vi "ReadTables1212(Host).vi"(0 "resource name":T1="RIO0" caption="RIO Device", 1 "Degree Offset":u16, 2 "NumSamples":u32=2048, 3 "DDS/ARB":bool=TRUE, 4 "Select Channel":u16(ring) items=["CH1", "CH2"], 5 "error in":errorcluster, 6 "FSampleDAC":dbl=2000000000.0 format="%#_6p", 7 "FoutDDS":dbl=85000000.0 format="%#_6p") -> (8 "error out":errorcluster)   [LabVIEW 2018]
uses:
  <vilib>/userdefined/High Color/nirio_resource_hc.ctl
  <vilib>/Utility/error.llb/Error Cluster From Error Code.vi
  <vilib>/rvi/errors/niLvFpgaAdjustHostInterfaceError.vi
  <vilib>/FPGAPlugInAG/Dynamic/niLvFpga_Close_Dynamic.vi
  <vilib>/rvi/interface/nirviReadWriteControl/nirviReadWriteControl.xnode
  <vilib>/rvi/interface/nirviCloseFPGA/nirviCloseFPGA.xnode
  NiFpgaLv.dll
  <vilib>/rvi/interface/Simulation/niFpgaSimulationCallBeginRW.vi
panel:
  out "FPGA Interface Out":refnum<k20>
  in  "FPGA Interface In":refnum<k20>
  in  "FLEX RIO RESET":bool
  in  "StartAddress8_CH1":u32=2920577760
  in  "StartAddress7_CH1":u32=2738041650
  in  "StartAddress6_CH1":u32=2555505540
  in  "StartAddress5_CH1":u32=2372969430
  in  "StartAddress4_CH1":u32=2190433320
  in  "StartAddress3_CH1":u32=2007897210
  in  "StartAddress2_CH1":u32=1825361100
  in  "StartAddress1_CH1":u32=1642824990
  in  "StartAddress8_CH0":u32=1460288880
  in  "StartAddress7_CH0":u32=1277752770
  in  "StartAddress6_CH0":u32=1095216660
  in  "StartAddress5_CH0":u32=912680550
  in  "StopAddress8_CH1":u32=2047
  out "Data16":fxp<+,14,14>=2760.0
  out "Data15":fxp<+,14,14>=3625.0
  in  "StopAddress7_CH1":u32=2046
  out "Data14":fxp<+,14,14>=4813.0
  in  "StopAddress6_CH1":u32=2045
  out "Data13":fxp<+,14,14>=6240.0
  in  "StopAddress5_CH1":u32=2044
  out "Data12":fxp<+,14,14>=7806.0
  in  "StopAddress4_CH1":u32=2043
  out "Data11":fxp<+,14,14>=9399.0
  in  "StopAddress3_CH1":u32=2042
  out "Data10":fxp<+,14,14>=10906.0
  out "Data9":fxp<+,14,14>=12221.0
  in  "StopAddress1_CH1":u32=2040
  in  "StopAddress2_CH1":u32=2041
  out "Data5":fxp<+,14,14>=14030.0
  in  "StopAddress5_CH0":u32=2036
  out "Data6":fxp<+,14,14>=14189.0
  in  "StopAddress6_CH0":u32=2037
  out "Data7":fxp<+,14,14>=13923.0
  in  "StopAddress7_CH0":u32=2038
  out "Data8":fxp<+,14,14>=13251.0
  in  "StopAddress8_CH0":u32=2039
  out "Data4":fxp<+,14,14>=13457.0
  out "Data3":fxp<+,14,14>=12512.0
  in  "StopAddress4_CH0":u32=2035
  in  "StopAddress3_CH0":u32=2034
  in  "StartAddress4_CH0":u32=730144440
  in  "StartAddress3_CH0":u32=547608330
  in  "Increment":u32=16 format="%.0x"
  in  "StartAddress2_CH0":u32=365072220
  in  "StopAddress2_CH0":u32=2033
  in  "StopAddress1_CH0":u32=2032
  in  "StartAddress1_CH0":u32=182536110
  in  "FPGA RESET":bool
  in  "IO Module\\trig_out":bool
  out "IO Module\\lockedfast":bool=TRUE
  out "IO Module\\trig_in":bool
  out "Data2":fxp<+,14,14>=11261.0
  out "Data1":fxp<+,14,14>=9792.0
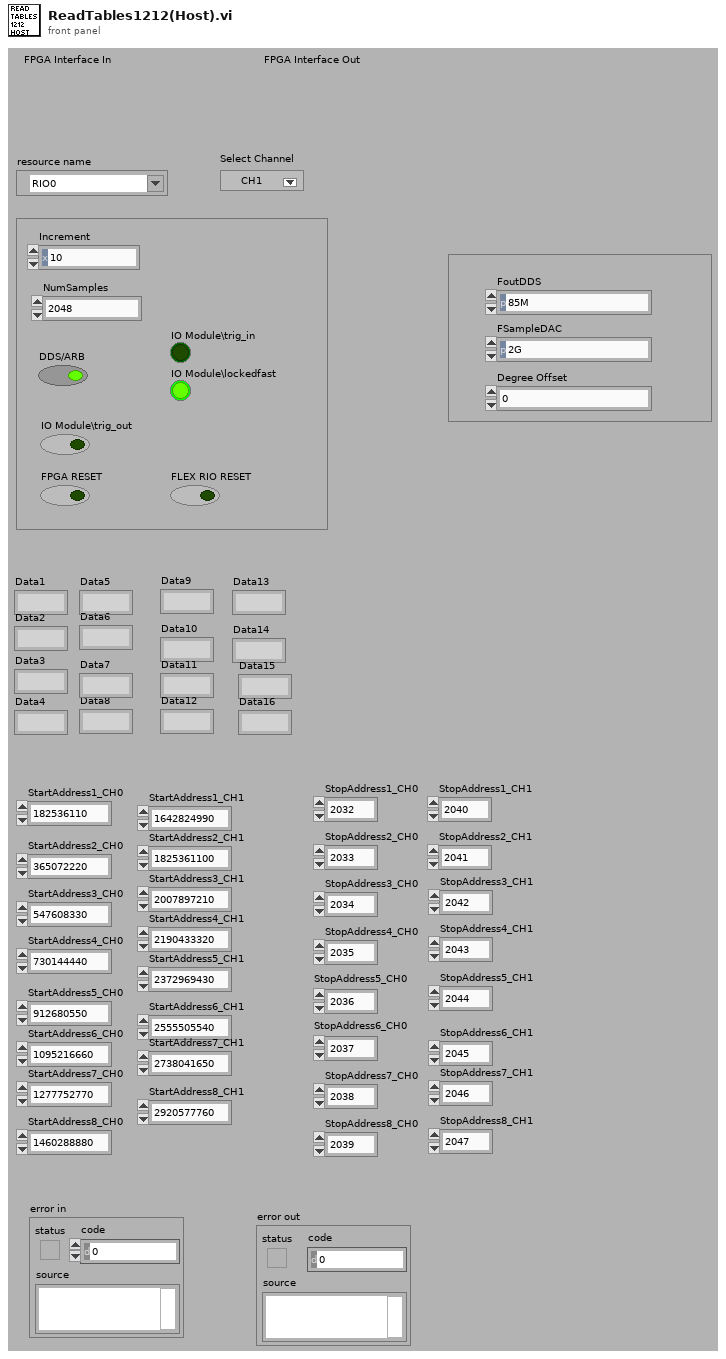
[diagram p1: front panel]
types:
  T1 = typedef "nirio_resource_hc.ctl" = tag
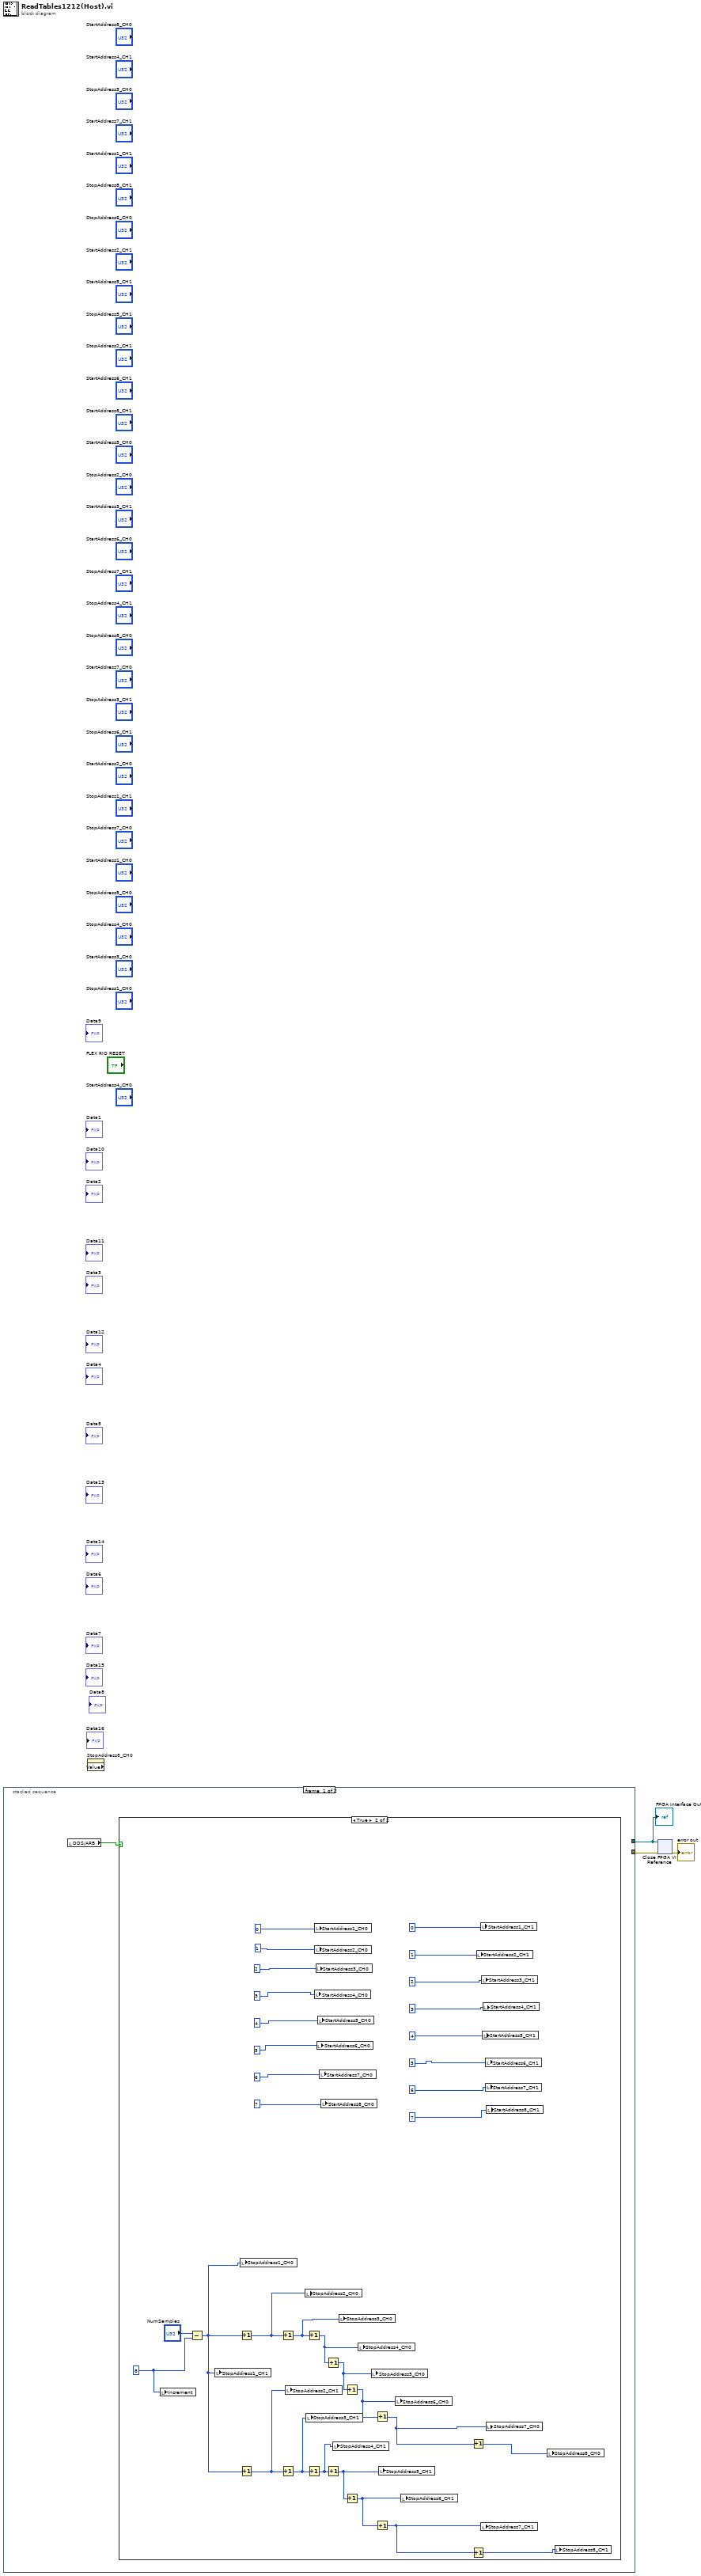
[diagram p0: block diagram]
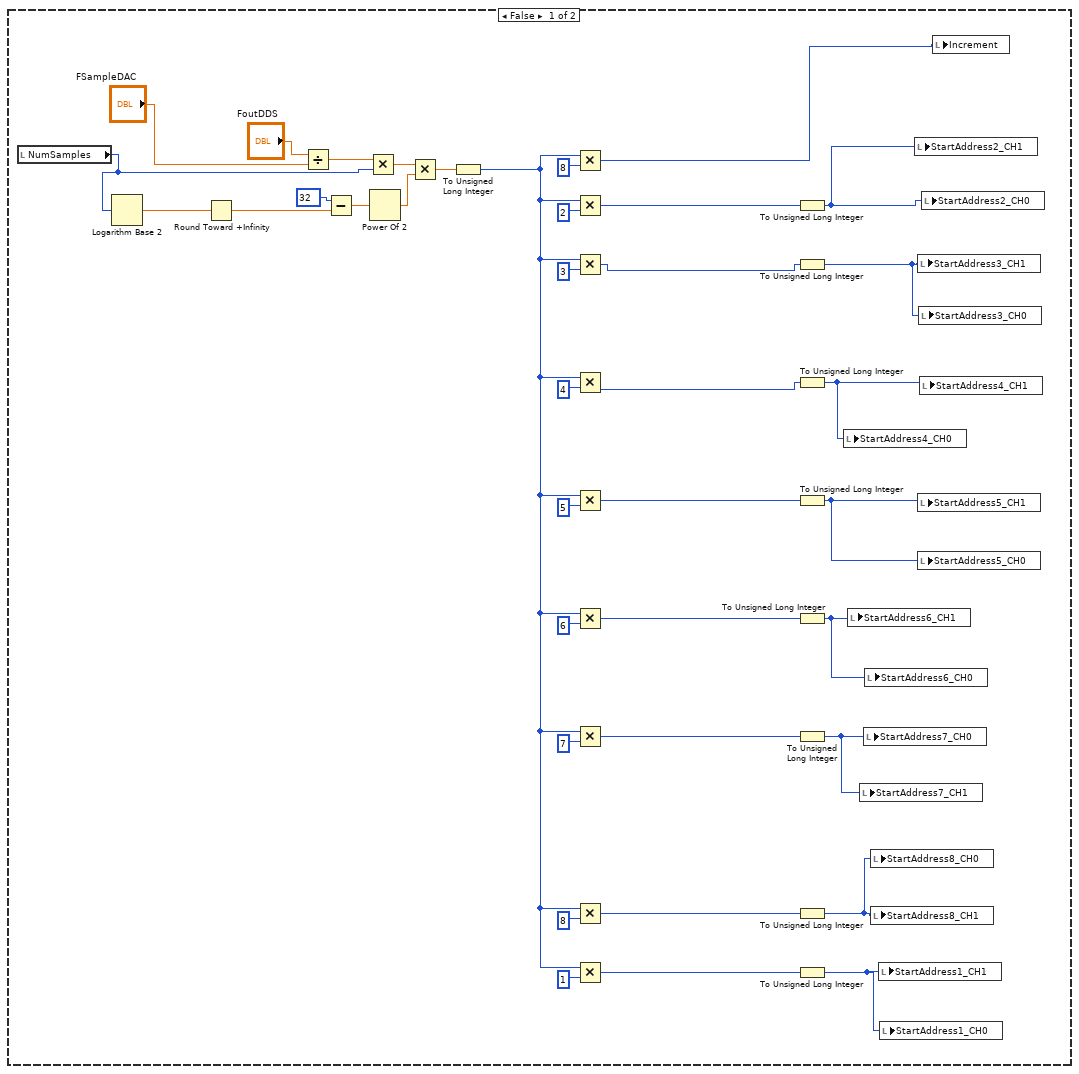
[diagram p2: hidden frame]
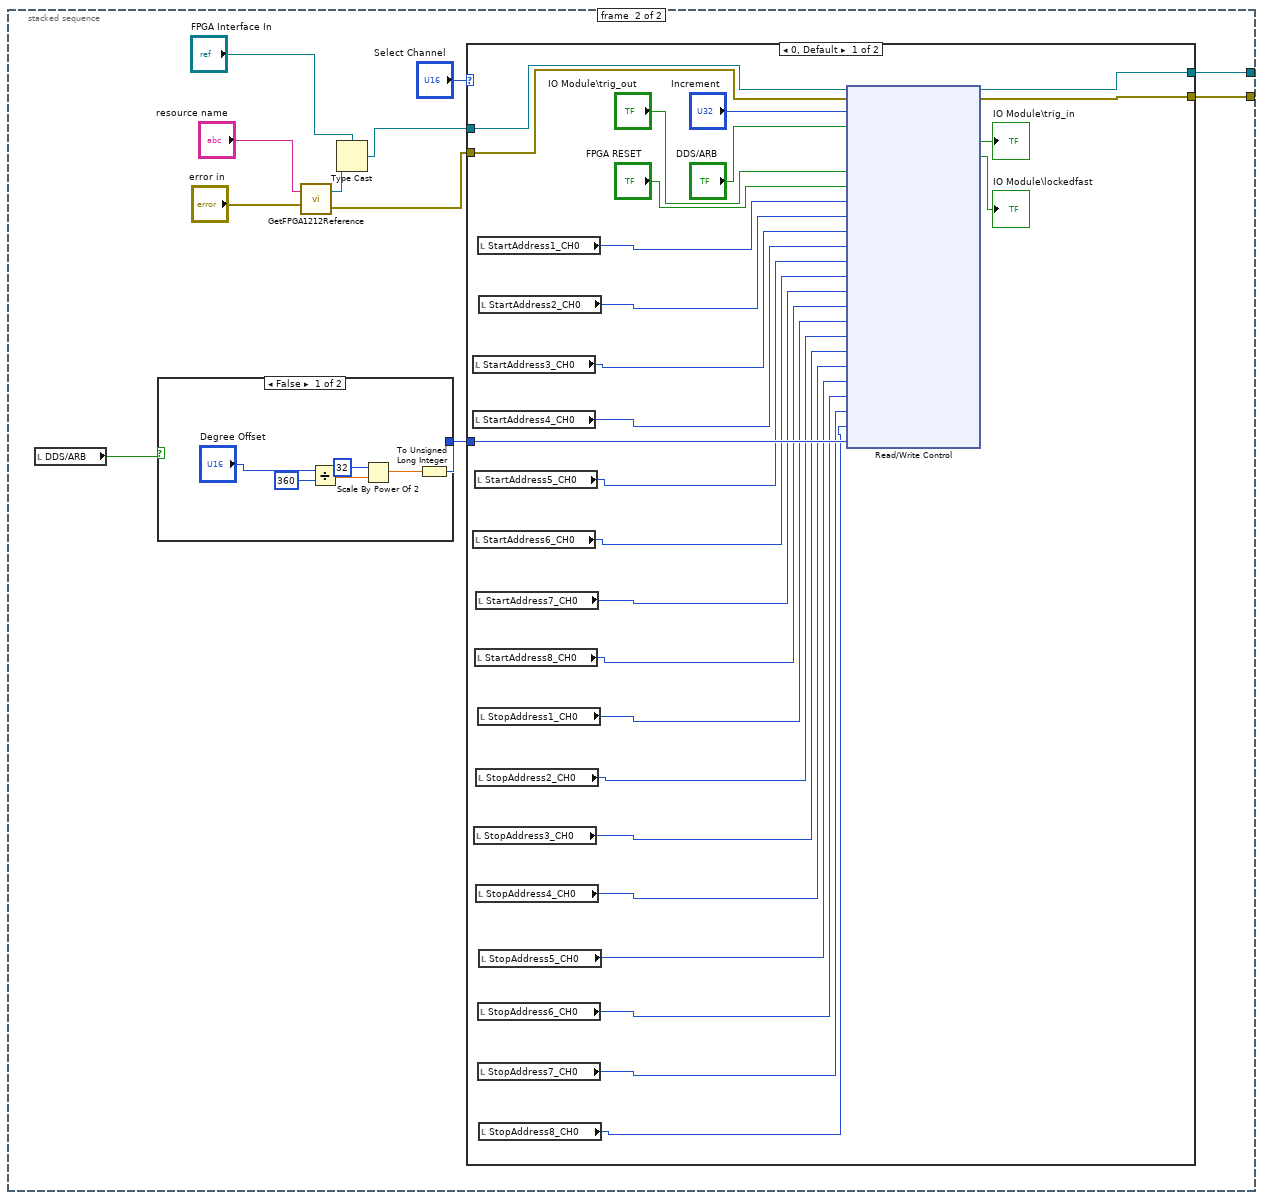
[diagram p3: hidden frame]
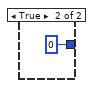
[diagram p4: hidden frame]
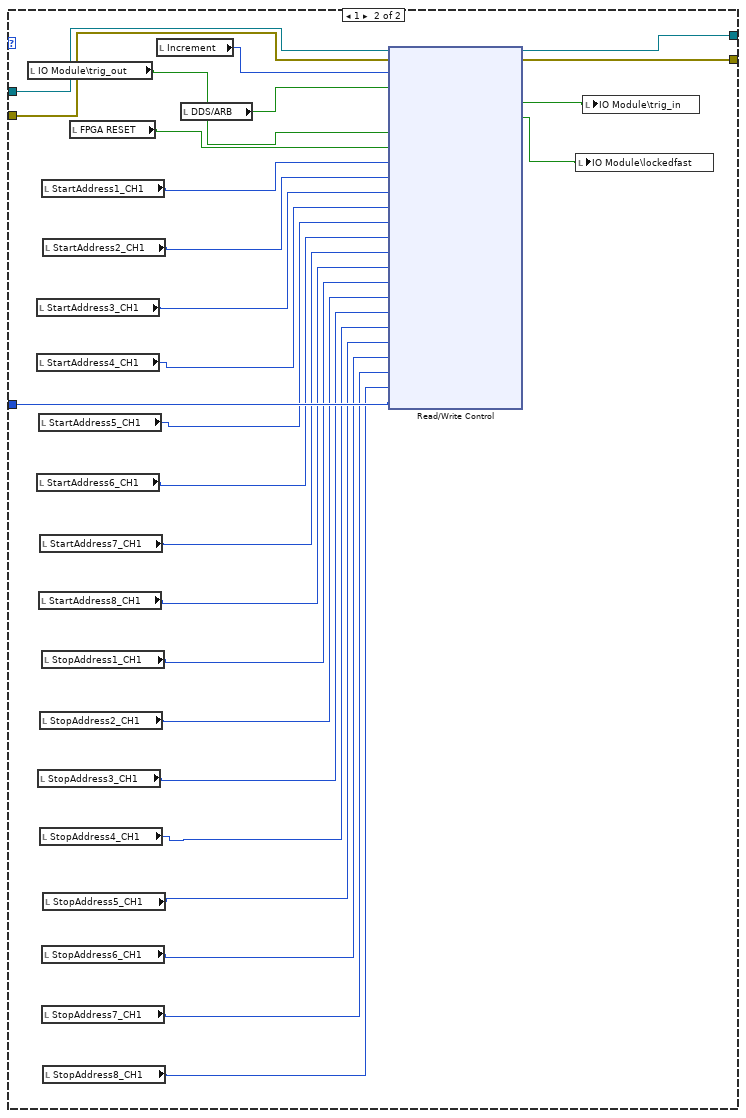
[diagram p5: hidden frame]
diagram:
  n1 = stacked-sequence {
    tunnel: [_ w86] -> w2
    tunnel: [_ w85] -> w1
    frame #0 {
      n2 = local read "DDS/ARB"() -> (w4:bool)
      n3 = case shown="True" w4 {
        frame False {
          n4 = local read "NumSamples"() -> (w14:u32)
          n5 = Logarithm Base 2(1:w14) -> (0:w26:dbl)
          n6 = Round Toward +Infinity(x=w26) -> (ceil(x): smallest int >= x=w25:dbl)
          n7 = Divide(x="FoutDDS", y="FSampleDAC") -> (x/y=w35:dbl)
          n8 = Subtract(x=u32 32, y=w25) -> (x-y=w28:dbl)
          n9 = Multiply(x=w35, y=w14) -> (x*y=w34:dbl)
          n10 = Power Of 2(x=w28) -> (2^x=w27:dbl)
          n11 = Multiply(x=w34, y=w27) -> (x*y=w33:dbl)
          n12 = To Unsigned Long Integer(number=w33) -> (unsigned 32bit integer=w23:u32)
          n13 = Multiply(x=w23, y=u32 8) -> (x*y=w13:u32)
          n14 = Multiply(x=w23, y=u32 2) -> (x*y=w22:u32)
          n15 = Multiply(x=w23, y=u32 3) -> (x*y=w21:u32)
          n16 = Multiply(x=w23, y=u32 4) -> (x*y=w20:u32)
          n17 = Multiply(x=w23, y=u32 5) -> (x*y=w19:u32)
          n18 = Multiply(x=w23, y=u32 6) -> (x*y=w18:u32)
          n19 = Multiply(x=w23, y=u32 7) -> (x*y=w17:u32)
          n20 = Multiply(x=w23, y=u32 8) -> (x*y=w16:u32)
          n21 = Multiply(x=w23, y=u32 1) -> (x*y=w15:u32)
          n22 = To Unsigned Long Integer(number=w22) -> (unsigned 32bit integer=w12:u32)
          n23 = To Unsigned Long Integer(number=w21) -> (unsigned 32bit integer=w11:u32)
          n24 = To Unsigned Long Integer(number=w20) -> (unsigned 32bit integer=w10:u32)
          n25 = To Unsigned Long Integer(number=w19) -> (unsigned 32bit integer=w9:u32)
          n26 = To Unsigned Long Integer(number=w18) -> (unsigned 32bit integer=w8:u32)
          n27 = To Unsigned Long Integer(number=w17) -> (unsigned 32bit integer=w7:u32)
          n28 = To Unsigned Long Integer(number=w16) -> (unsigned 32bit integer=w6:u32)
          n29 = To Unsigned Long Integer(number=w15) -> (unsigned 32bit integer=w5:u32)
          n30 = local write "StartAddress4_CH0"(w10) -> ()
          n31 = local write "StartAddress6_CH1"(w8) -> ()
          n32 = local write "StartAddress7_CH1"(w7) -> ()
          n33 = local write "StartAddress7_CH0"(w7) -> ()
          n34 = local write "StartAddress6_CH0"(w8) -> ()
          n35 = local write "StartAddress8_CH0"(w6) -> ()
          n36 = local write "StartAddress8_CH1"(w6) -> ()
          n37 = local write "StartAddress1_CH1"(w5) -> ()
          n38 = local write "StartAddress1_CH0"(w5) -> ()
          n39 = local write "StartAddress2_CH1"(w12) -> ()
          n40 = local write "StartAddress3_CH1"(w11) -> ()
          n41 = local write "StartAddress5_CH1"(w9) -> ()
          n42 = local write "StartAddress5_CH0"(w9) -> ()
          n43 = local write "StartAddress3_CH0"(w11) -> ()
          n44 = local write "StartAddress4_CH1"(w10) -> ()
          n45 = local write "StartAddress2_CH0"(w12) -> ()
          n46 = local write "Increment"(w13) -> ()
        }
        frame True {
          w58 = u32 8 ("y")
          n47 = local write "Increment"(w58) -> ()
          n48 = Subtract(x="NumSamples", y=w58) -> (x-y=w50:u32)
          n49 = local write "StopAddress1_CH1"(w50) -> ()
          n50 = Increment(x=w50) -> (x+1=w51:u32)
          n51 = Increment(x=w50) -> (x+1=w49:u32)
          n52 = local write "StopAddress1_CH0"(w50) -> ()
          n53 = Increment(x=w51) -> (x+1=w52:u32)
          n54 = Increment(x=w49) -> (x+1=w48:u32)
          n55 = local write "StopAddress2_CH1"(w49) -> ()
          n56 = local write "StopAddress2_CH0"(w51) -> ()
          n57 = local write "StopAddress3_CH1"(w48) -> ()
          n58 = Increment(x=w52) -> (x+1=w53:u32)
          n59 = Increment(x=w48) -> (x+1=w47:u32)
          n60 = local write "StartAddress4_CH0"(u32 3 ("StartAddress1")) -> ()
          n61 = local write "StartAddress1_CH0"(u32 0 ("StartAddress1")) -> ()
          n62 = local write "StartAddress2_CH0"(u32 1 ("StartAddress1")) -> ()
          n63 = local write "StartAddress3_CH0"(u32 2 ("StartAddress1")) -> ()
          n64 = local write "StartAddress6_CH0"(u32 5 ("StartAddress1")) -> ()
          n65 = local write "StartAddress5_CH0"(u32 4 ("StartAddress1")) -> ()
          n66 = local write "StartAddress7_CH0"(u32 6 ("StartAddress1")) -> ()
          n67 = local write "StartAddress8_CH0"(u32 7 ("StartAddress1")) -> ()
          n68 = Increment(x=w53) -> (x+1=w54:u32)
          n69 = Increment(x=w47) -> (x+1=w46:u32)
          n70 = local write "StopAddress4_CH1"(w47) -> ()
          n71 = local write "StopAddress3_CH0"(w52) -> ()
          n72 = Increment(x=w54) -> (x+1=w55:u32)
          n73 = Increment(x=w46) -> (x+1=w45:u32)
          n74 = local write "StopAddress4_CH0"(w53) -> ()
          n75 = local write "StopAddress5_CH0"(w54) -> ()
          n76 = Increment(x=w55) -> (x+1=w56:u32)
          n77 = Increment(x=w45) -> (x+1=w44:u32)
          n78 = local write "StopAddress5_CH1"(w46) -> ()
          n79 = local write "StopAddress6_CH0"(w55) -> ()
          n80 = local write "StopAddress6_CH1"(w45) -> ()
          n81 = Increment(x=w56) -> (x+1=w57:u32)
          n82 = Increment(x=w44) -> (x+1=w43:u32)
          n83 = local write "StartAddress2_CH1"(u32 1 ("StartAddress1")) -> ()
          n84 = local write "StartAddress1_CH1"(u32 0 ("StartAddress1")) -> ()
          n85 = local write "StopAddress7_CH1"(w44) -> ()
          n86 = local write "StartAddress3_CH1"(u32 2 ("StartAddress1")) -> ()
          n87 = local write "StartAddress5_CH1"(u32 4 ("StartAddress1")) -> ()
          n88 = local write "StartAddress4_CH1"(u32 3 ("StartAddress1")) -> ()
          n89 = local write "StartAddress6_CH1"(u32 5 ("StartAddress1")) -> ()
          n90 = local write "StartAddress7_CH1"(u32 6 ("StartAddress1")) -> ()
          n91 = local write "StopAddress7_CH0"(w56) -> ()
          n92 = local write "StartAddress8_CH1"(u32 7 ("StartAddress1")) -> ()
          n93 = local write "StopAddress8_CH0"(w57) -> ()
          n94 = local write "StopAddress8_CH1"(w43) -> ()
        }
      }
    }
    frame #1 {
      n95 = local read "DDS/ARB"() -> (w76:bool)
      n96 = case shown="False" w76 {
        tunnel: [w87 u32 0] -> w83
        frame False {
          n97 = Divide(x="Degree Offset", y=u16 360) -> (x/y=w90:dbl)
          n98 = Scale By Power Of 2(n=32, x=w90) -> (x*2^n=w88:dbl)
          n99 = To Unsigned Long Integer(number=w88) -> (unsigned 32bit integer=w87:u32)
        }
        frame True {
        }
      }
      n100 = call "GetFPGA1212Reference.vi"("error in"="error in", "RIO Device IN"="resource name") -> ("error out"=w78:errorcluster, "FPGA VI Reference Out"=w82:refnum<k20>)
      n101 = Type Cast(type="FPGA Interface In", x=w82) -> (*(type *) &x=w77:refnum<k20>)
      n102 = case shown="0, Default" "Select Channel" {
        tunnel: [w116 w147] -> w86
        tunnel: w78 -> [w115 w146]
        tunnel: w77 -> [w114 w143]
        tunnel: [w113 w145] -> w85
        tunnel: w83 -> [w111 w144]
        frame 0, Default {
          n103 = local read "StartAddress3_CH0"() -> (w107:u32)
          n104 = local read "StartAddress4_CH0"() -> (w106:u32)
          n105 = local read "StartAddress6_CH0"() -> (w104:u32)
          n106 = local read "StopAddress3_CH0"() -> (w99:u32)
          n107 = local read "StartAddress5_CH0"() -> (w105:u32)
          n108 = local read "StartAddress8_CH0"() -> (w102:u32)
          n109 = local read "StartAddress7_CH0"() -> (w103:u32)
          n110 = local read "StopAddress2_CH0"() -> (w100:u32)
          n111 = local read "StopAddress4_CH0"() -> (w98:u32)
          n112 = local read "StartAddress1_CH0"() -> (w109:u32)
          n113 = local read "StopAddress1_CH0"() -> (w101:u32)
          n114 = local read "StopAddress6_CH0"() -> (w96:u32)
          n115 = local read "StopAddress7_CH0"() -> (w95:u32)
          n116 = local read "StartAddress2_CH0"() -> (w108:u32)
          n117 = local read "StopAddress5_CH0"() -> (w97:u32)
          n118 = local read "StopAddress8_CH0"() -> (w94:u32)
          n119 = xnode "Read/Write Control"("FPGA VI Reference In"=w114, "error in"=w115, "Increment_CH0"="Increment", "DDS/ARB CH0"="DDS/ARB", "IO Module\\trig_out"="IO Module\\trig_out", "SysReset"="FPGA RESET", "StartAddress1_CH0"=w109, "StartAddress2_CH0"=w108, "StartAddress3_CH0"=w107, "StartAddress4_CH0"=w106, "StartAddress5_CH0"=w105, "StartAddress6_CH0"=w104, "StartAddress7_CH0"=w103, "StartAddress8_CH0"=w102, "StopAddress1_CH0"=w101, "StopAddress2_CH0"=w100, "StopAddress3_CH0"=w99, "StopAddress4_CH0"=w98, "StopAddress5_CH0"=w97, "StopAddress6_CH0"=w96, "StopAddress7_CH0"=w95, "StopAddress8_CH0"=w94, "Offset_CH0"=w111) -> ("FPGA VI Reference Out"=w113:refnum<k20>, "error out"=w116:errorcluster, "IO Module\\trig_in"=→"IO Module\\trig_in":bool, "IO Module\\lockedfast"=→"IO Module\\lockedfast":bool)
        }
        frame 1 {
          n120 = local read "IO Module\\trig_out"() -> (w141:bool)
          n121 = local read "StartAddress3_CH1"() -> (w136:u32)
          n122 = local read "StartAddress4_CH1"() -> (w135:u32)
          n123 = local read "StartAddress6_CH1"() -> (w133:u32)
          n124 = local read "StopAddress3_CH1"() -> (w128:u32)
          n125 = local read "StartAddress5_CH1"() -> (w134:u32)
          n126 = local read "StartAddress8_CH1"() -> (w131:u32)
          n127 = local read "StartAddress7_CH1"() -> (w132:u32)
          n128 = local read "StopAddress2_CH1"() -> (w129:u32)
          n129 = local read "StopAddress4_CH1"() -> (w127:u32)
          n130 = local read "StartAddress1_CH1"() -> (w138:u32)
          n131 = local read "StopAddress1_CH1"() -> (w130:u32)
          n132 = local read "StopAddress6_CH1"() -> (w125:u32)
          n133 = local read "StopAddress7_CH1"() -> (w124:u32)
          n134 = local read "StartAddress2_CH1"() -> (w137:u32)
          n135 = local read "StopAddress5_CH1"() -> (w126:u32)
          n136 = local read "StopAddress8_CH1"() -> (w123:u32)
          n137 = local read "FPGA RESET"() -> (w142:bool)
          n138 = local read "Increment"() -> (w139:u32)
          n139 = local read "DDS/ARB"() -> (w140:bool)
          n140 = xnode "Read/Write Control"("FPGA VI Reference In"=w143, "error in"=w146, "Increment_CH1"=w139, "DDS/ARB CH1"=w140, "IO Module\\trig_out"=w141, "SysReset"=w142, "StartAddress1_CH1"=w138, "StartAddress2_CH1"=w137, "StartAddress3_CH1"=w136, "StartAddress4_CH1"=w135, "StartAddress5_CH1"=w134, "StartAddress6_CH1"=w133, "StartAddress7_CH1"=w132, "StartAddress8_CH1"=w131, "StopAddress1_CH1"=w130, "StopAddress2_CH1"=w129, "StopAddress3_CH1"=w128, "StopAddress4_CH1"=w127, "StopAddress5_CH1"=w126, "StopAddress6_CH1"=w125, "StopAddress7_CH1"=w124, "StopAddress8_CH1"=w123, "Offset_CH1"=w144) -> ("FPGA VI Reference Out"=w145:refnum<k20>, "error out"=w147:errorcluster, "IO Module\\trig_in"=w121:bool, "IO Module\\lockedfast"=w122:bool)
          n141 = local write "IO Module\\lockedfast"(w122) -> ()
          n142 = local write "IO Module\\trig_in"(w121) -> ()
        }
      }
    }
  }
  "FPGA Interface Out" <- w1
  n143 = property on="StopAddress8_CH0" class="DigNum (strict)" props=["Value"]() -> ()  [unwired: 2 in, 3 out]
  n144 = xnode "Close FPGA VI Reference"("FPGA VI Reference In"=w1, "error in"=w2) -> ("error out"=→"error out":errorcluster)
